vi "Teleop.vi"(10 "Match Info":T2={"Autonomous Elapsed Seconds"=0.0, "TeleOp Elapsed Seconds"=0.0, "Disabled Elapsed Seconds"=0.0, "Visited Autonomous"=FALSE, "Visited TeleOp"=FALSE, "Visited Disabled"=FALSE, "Autonomous Settings"={"Autonomous Style"=enum."Independent", "VI Refnum"=refnum}}, 11 "Call Context":T3) -> ()   [LabVIEW 2015]
doc: "This VI is called for each TeleOp packet received from the DS where the robot is not disabled. It is often used to read from the joysticks and update I/O or to update setpoints for timed control loops. It should complete and return within 20 milliseconds or it may miss DS packets."
uses:
  <vilib>/Rock Robotics/WPI/DriverStation/WPI_DriverStationDerivedRobotMode.ctl
  <vilib>/Rock Robotics/WPI/DriverStation/WPI_DriverStationMatch Info.ctl
  <vilib>/Rock Robotics/WPI/Utilities/WPI_GetSetVariantRefNum.vi
  <vilib>/Rock Robotics/Network Tables/NT Write Boolean Array.vi
  <vilib>/Rock Robotics/Network Tables/NT Write Numeric Array.vi
  <vilib>/Rock Robotics/Network Tables/NT Read Boolean.vi
  <vilib>/Rock Robotics/Network Tables/NT Read Number.vi
  Robot Global Data.vi
  <vilib>/Rock Robotics/Network Tables/NT Write Number.vi
  <vilib>/Rock Robotics/WPI/RobotDrive/WPI_RobotDriveArcadeDrive_Standard(NoSaturation).vi
panel:
  in  "Winch Lock":bool
  out "Ladder Up Start Time":u32
  in  "LadderStateMachine":i32
  out "Accelerations":T1
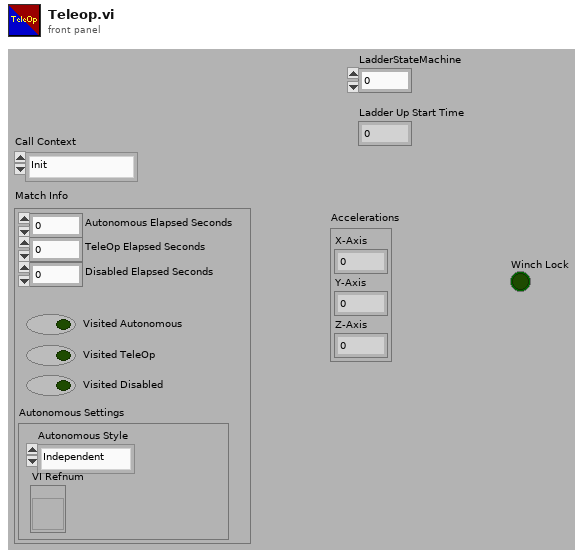
[diagram p1: front panel]
types:
  T1 = cluster{"X-Axis":dbl, "Y-Axis":dbl, "Z-Axis":dbl}
  T2 = typedef "WPI_DriverStationMatch Info.ctl" = cluster{"Autonomous Elapsed Seconds":dbl, "TeleOp Elapsed Seconds":dbl, "Disabled Elapsed Seconds":dbl, "Visited Autonomous":bool, "Visited TeleOp":bool, "Visited Disabled":bool, "Autonomous Settings":cluster{"Autonomous Style":enum16{"Iterative", "Independent"}, "VI Refnum":refnum<vi>}}
  T3 = typedef "WPI_DriverStationDerivedRobotMode.ctl" = enum16{"Init", "Execute", "Stop"}
  T4 = typedef "WPI_RobotDriveDevRef.ctl" = cluster{"DevStatus":errorcluster, "Motors[]":T5[], "Square Inputs":bool, "Max Output":dbl}
  T5 = typedef "WPI_MotorControlDeviceRef.ctl" = cluster{"DeviceStatus":errorcluster, "Type":T6, "PWM":cluster{"PWM Channel":T7, "DeadBand":T8}, "CAN":cluster{"Device Number":u8, "Control Mode":T9, "Semaphore":T10, "Max Vout":dbl, "TalonSRX Control Mode":T11}, "Invert":bool}
  T6 = typedef "WPI_MotorControlType.ctl" = enum16{"PWM", "CAN", "CANTalonSRX"}
  T7 = typedef "FPGA_DIOPWMChannel.ctl" = enum8{"PWM 0", "PWM 1", "PWM 2", "PWM 3", "PWM 4", "PWM 5", "PWM 6", "PWM 7", "PWM 8", "PWM 9", "PWM MXP 0", "PWM MXP 1", "PWM MXP 2", "PWM MXP 3", "PWM MXP 4", "PWM MXP 5", "PWM MXP 6", "PWM MXP 7", "PWM MXP 8", "PWM MXP 9", "Invalid"}
  T8 = typedef "WPI_PWMDeadband.ctl" = cluster{"Name":string, "maxPositivePwm":i32, "minPositivePwm":i32, "centerPwm":i32, "maxNegativePwm":i32, "minNegativePwm":i32, "angularRange":u16}
  T9 = typedef "WPI_CANJaguar_ControlMode.ctl" = enum8{"Percent VBus", "Current", "Speed", "Position", "Voltage"}
  T10 = typedef "Semaphore RefNum" = refnum<k1>
  T11 = typedef "WPI_CANTalonSRX_APIControlMode.ctl" = enum8{"Percent VBus", "Speed", "Position", "Slave", "Unchanged / Invalid", "Voltage Compensation", "Current", "Motion Profile"}
  T12 = typedef "WPI_JoystickDevRef.ctl" = cluster{"Device":T13}
  T13 = typedef "WPI_JoystickDeviceEnum.ctl" = enum16{"USB 0", "USB 1", "USB 2", "USB 3", "USB 4", "USB 5"}
  T14 = typedef "WPI_DigitalInputDevRef.ctl" = cluster{"DevStatus":errorcluster, "DIO Channel":T15}
  T15 = typedef "FPGA_DIOChannel.ctl" = enum8{"DIO 0", "DIO 1", "DIO 2", "DIO 3", "DIO 4", "DIO 5", "DIO 6", "DIO 7", "DIO 8", "DIO 9", "DIO MXP 0", "DIO MXP 1", "DIO MXP 2", "DIO MXP 3", "DIO MXP 4", "DIO MXP 5", "DIO MXP 6", "DIO MXP 7", "DIO MXP 8", "DIO MXP 9", "DIO MXP 10", "DIO MXP 11", "DIO MXP 12", "DIO MXP 13", "DIO MXP 14", "DIO MXP 15", "Invalid"}
  T16 = typedef "WPI_AccelerometerDevRef.ctl" = cluster{"DevStatus":errorcluster, "Scaling":T17, "Analog Channels":T18, "I2C Bus":T20, "SPI Bus":T21, "Accel Range":T22, "ADXL Axes":T23, "Handle":i32, "Device Address":u8, "Accel Type":enum16{"Analog", "ADXL345 I2C", "ADXL345 SPI", "Internal", "ADXL362 SPI"}}
  T17 = typedef "WPI_AccelerometerScaling.ctl" = cluster{"Gain (VoltsPerG)":dbl, "Center Voltage":dbl}
  T18 = typedef "WPI_AccelerometerAnalogChannels.ctl" = cluster{"X-Axis":T19, "Y-Axis":T19, "Z-Axis":T19}
  T19 = typedef "FPGA_AIChannel.ctl" = enum8{"AI 0", "AI 1", "AI 2", "AI 3", "AI MXP 0", "AI MXP 1", "AI MXP 2", "AI MXP 3", "Invalid"}
  T20 = typedef "i2c_bus.ctl" = enum16{"I2C On-Board", "I2C MXP", "Invalid"}
  T21 = typedef "spi_bus.ctl" = enum16{"SPI On-Board, CS0", "SPI On-Board, CS1", "SPI On-Board, CS2", "SPI On-Board, CS3", "SPI MXP", "Invalid"}
  T22 = typedef "ADXL345 Range.ctl" = u8
  T23 = typedef "WPI_AccelerometerADXL345 Axes.ctl" = cluster{"X-Axis":bool, "Y-Axis":bool, "Z-Axis":bool}
  T24 = typedef "WPI_EncoderDevRef.ctl" = cluster{"DevStatus":errorcluster, "EncoderIndex":T25, "CounterIndex":T26, "DistancePerCount":dbl, "Decoding Type":T27}
  T25 = typedef "FPGA_EncoderIdx.ctl" = enum8{"Enc 0", "Enc 1", "Enc 2", "Enc 3", "Enc 4", "Enc 5", "Enc 6", "Enc 7", "Invalid"}
  T26 = typedef "FPGA_CounterCtrSystemIndex.ctl" = enum8{"Ctr 0", "Ctr 1", "Ctr 2", "Ctr 3", "Ctr 4", "Ctr 5", "Ctr 6", "Ctr 7", "Invalid"}
  T27 = typedef "WPI_EncoderType.ctl" = enum16{"1x", "2x", "4x"}
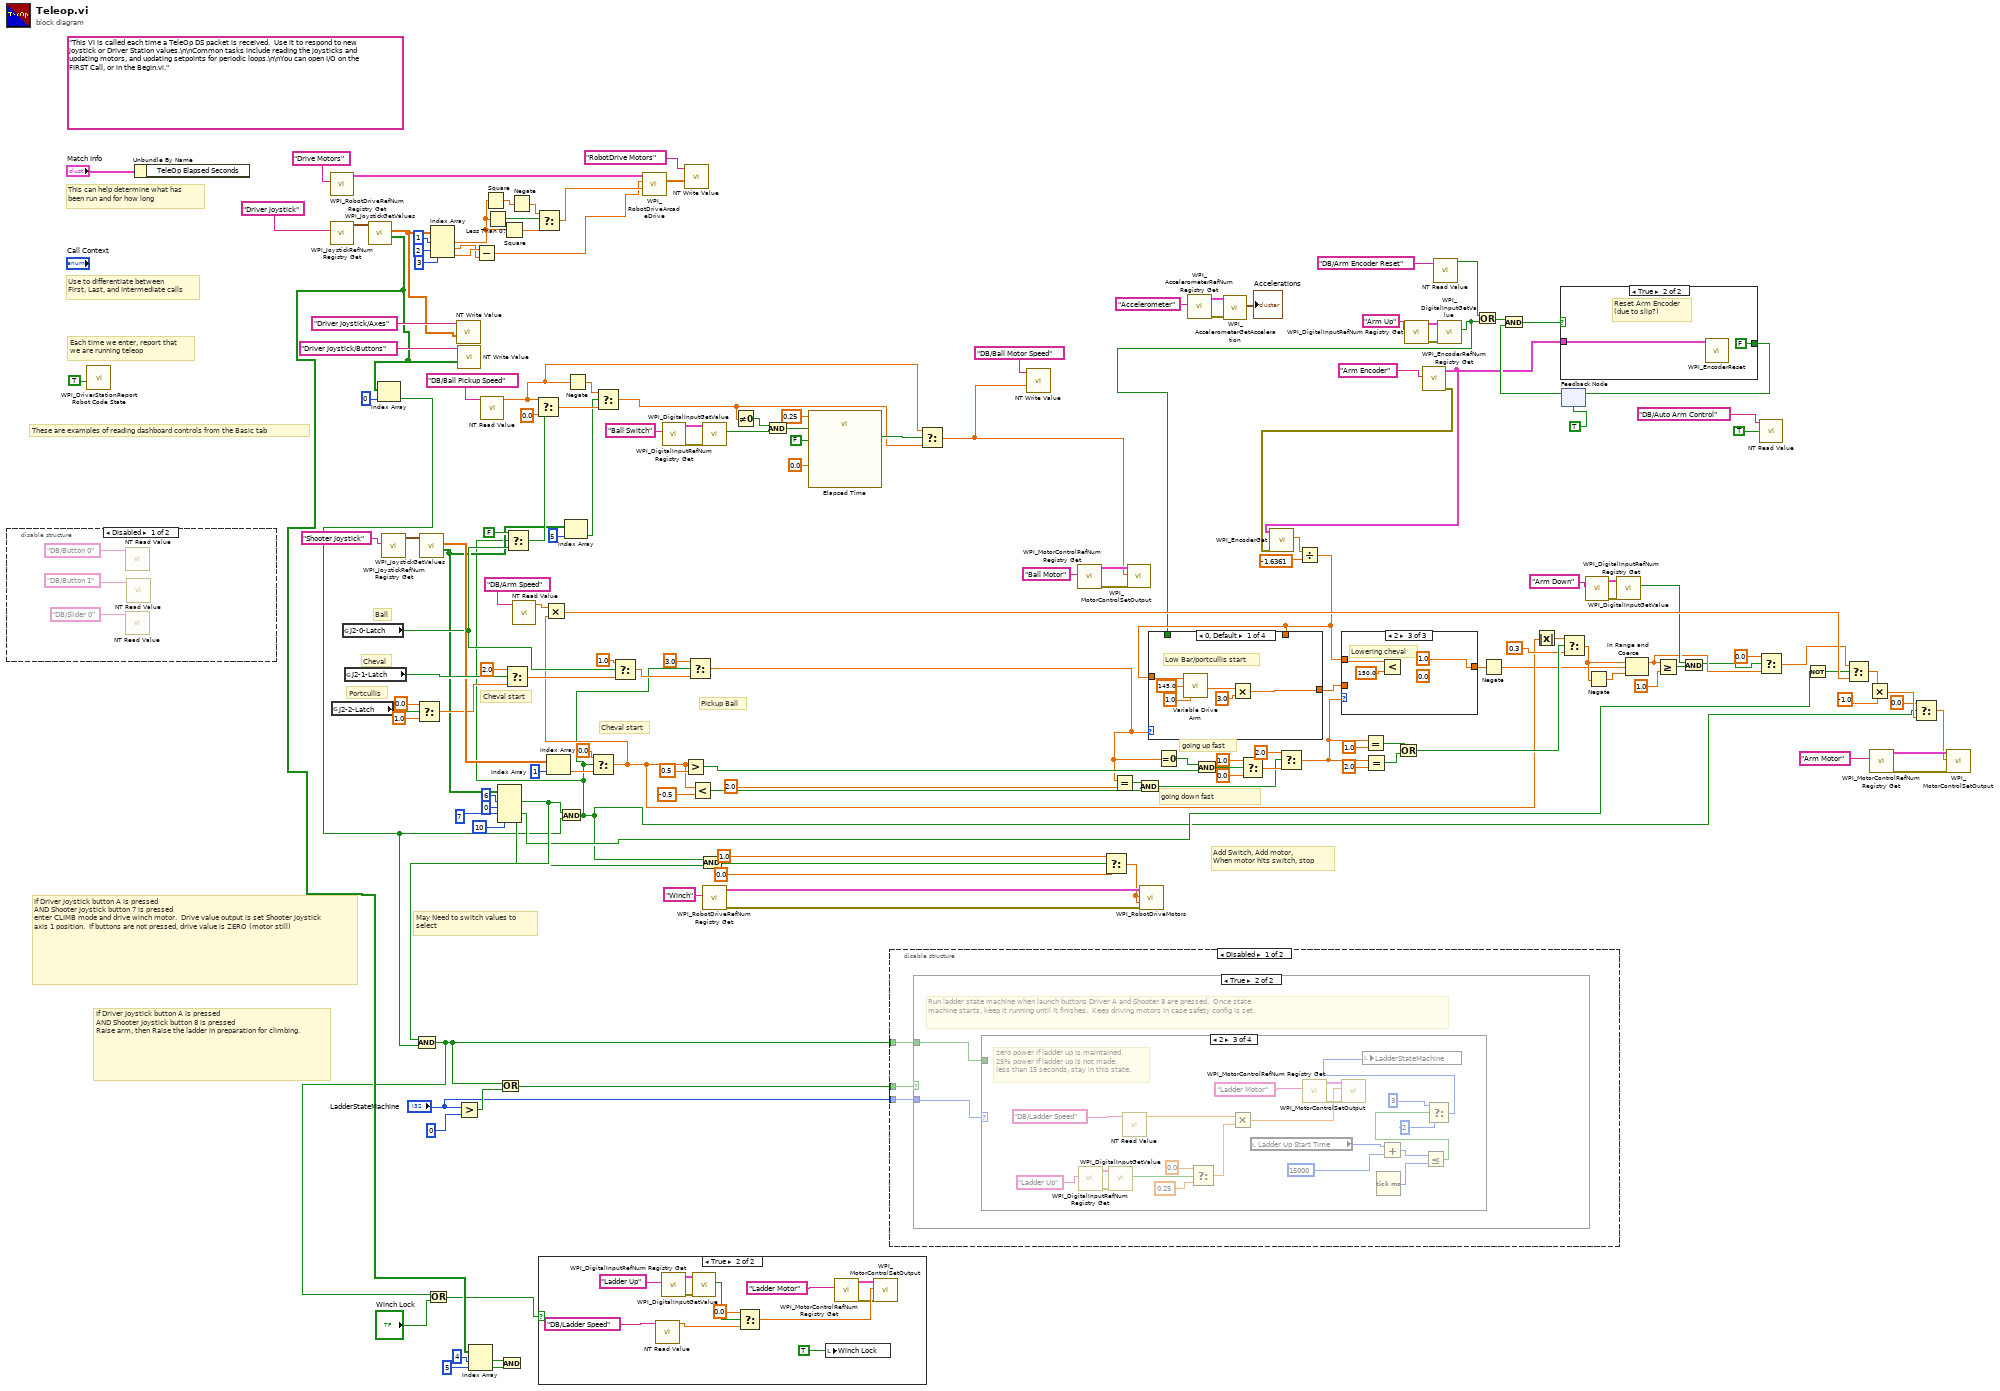
[diagram p0: block diagram]
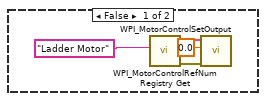
[diagram p2: hidden frame]
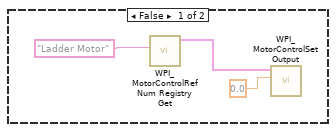
[diagram p3: hidden frame]
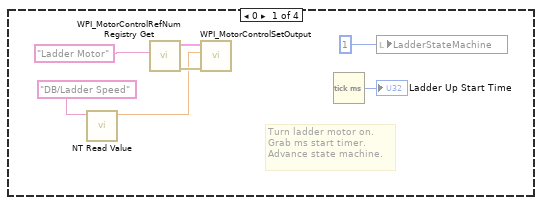
[diagram p4: hidden frame]
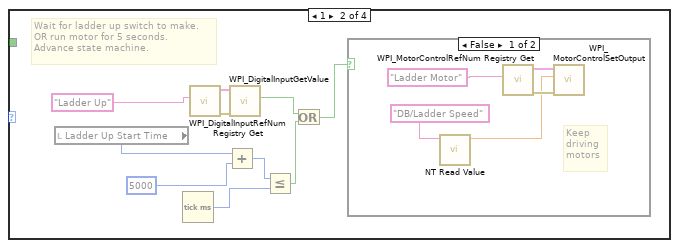
[diagram p5: hidden frame]
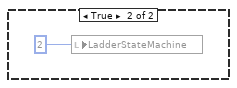
[diagram p6: hidden frame]
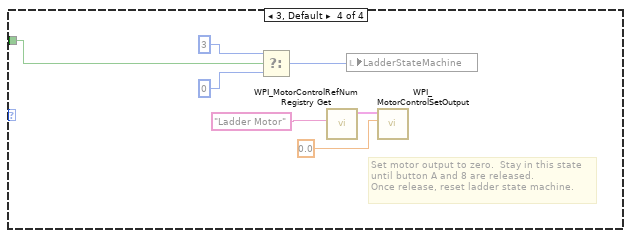
[diagram p7: hidden frame]
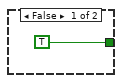
[diagram p9: hidden frame]
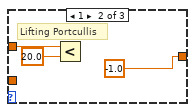
[diagram p12: hidden frame]
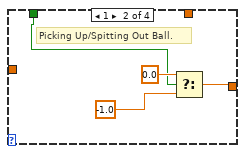
[diagram p13: hidden frame]
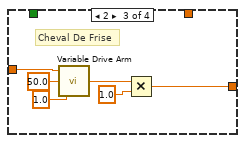
[diagram p14: hidden frame]
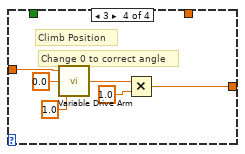
[diagram p15: hidden frame]
diagram:
  (unwired) "This VI is called each time a TeleOp DS packet is received.  Use it to respond to new joystick or Driver Station values.\n\nCommon tasks include reading the joysticks and updating motors, and updating setpoints for periodic loops.\n\nYou can open I/O on the FIRST Call, or in the Begin.vi."
  # "going up fast"
  # "going down fast"
  # "If Driver Joystick button A is pressed\nAND Shooter Joystick button 8 is pressed\nRaise arm, then Raise the ladder in preparation for climbing."
  # "If Driver Joystick button A is pressed\nAND Shooter Joystick button 7 is pressed\nenter CLIMB mode and drive winch motor.  Drive value output is set Shooter Joystick axis 1 position.  If buttons are not pressed, drive value is ZERO (motor still)"
  # "Add Switch, Add motor, \nWhen motor hits switch, stop"
  # "Portcullis"
  # "Ball"
  # "Cheval"
  # "May Need to switch values to \nselect"
  # "Cheval start"
  # "Pickup Ball"
  # "Cheval start"
  # "These are examples of reading dashboard controls from the Basic tab"
  # "Each time we enter, report that\nwe are running teleop"
  # "Use to differentiate between\nFirst, Last, and Intermediate calls"
  # "This can help determine what has\nbeen run and for how long"
  n1 = disable-structure shown="Disabled" {
    frame Disabled {
      n2 = call-poly <vilib>:"NT Read Value.vi"("Name"="DB/Button 0" ("refnum name")) -> ("Boolean"=w169:bool)  [unwired: 9 in, 1 out]
      n3 = call-poly <vilib>:"NT Read Value.vi"("Name"="DB/Slider 0" ("refnum name")) -> ("Numeric"=w171:dbl)  [unwired: 9 in, 1 out]
      n4 = call-poly <vilib>:"NT Read Value.vi"("Name"="DB/Button 1" ("refnum name")) -> ("Boolean"=w170:bool)  [unwired: 9 in, 1 out]
    }
    frame Enabled {
    }
  }
  n5 = call <vilib>:"WPI_DriverStationReport Robot Code State.vi"("TeleOp"=TRUE ("Autonomous")) -> ()  [unwired: 10 in, 1 out]
  n6 = Unbundle By Name("Match Info") -> ()  [unwired: 1 out]
  n7 = call <vilib>:"WPI_RobotDriveRefNum Registry Get.vi"("refnum name"="Drive Motors") -> ("RobotDriveDevRef"=w165:T4)  [unwired: 1 in, 9 out]
  n8 = call <vilib>:"WPI_JoystickRefNum Registry Get.vi"("refnum name"="Driver Joystick") -> ("JoystickDevRef"=w163:T12)  [unwired: 1 in, 9 out]
  n9 = global read "Robot Global Data.vi" "J2-2-Latch"() -> (w88:bool)
  n10 = global read "Robot Global Data.vi" "J2-0-Latch"() -> (w84:bool)
  n11 = global read "Robot Global Data.vi" "J2-1-Latch"() -> (w141:bool)
  n12 = call <vilib>:"WPI_JoystickGetValues.vi"("JoystickDevRef"=w163) -> ("Buttons"=w32:bool[], "Axes"=w153:dbl[])  [unwired: 6 in, 3 out]
  n13 = Index Array(array=w32, index=0) -> (element=w31:bool)
  n14 = call <vilib>:"WPI_JoystickRefNum Registry Get.vi"("refnum name"="Shooter Joystick") -> ("JoystickDevRef"=w152:T12)  [unwired: 1 in, 9 out]
  n15 = Select(t=0.0, s=w88, f=1.0) -> (s? t:f=w89:dbl)
  n16 = call <vilib>:"WPI_JoystickGetValues.vi"("JoystickDevRef"=w152) -> ("Buttons"=w56:bool[], "Axes"=w117:dbl[])  [unwired: 6 in, 3 out]
  n17 = Index Array(array=w153, index #1=1 ("index"), index #2=2 ("index"), index #3=3 ("index")) -> (element #1=w113:dbl, element #2=w110:dbl, element #3=w111:dbl)
  n18 = call-poly <vilib>:"NT Write Value.vi"("Numeric Array"=w153, "Name"="Driver Joystick/Axes") -> ()  [unwired: 9 in, 1 out]
  n19 = call-poly <vilib>:"NT Write Value.vi"("Boolean Array"=w32, "Name"="Driver Joystick/Buttons") -> ()  [unwired: 9 in, 1 out]
  n20 = Greater?(x="LadderStateMachine", y=0) -> (0:w69:bool)
  n21 = Index Array(array=w32, index #1=4 ("index"), index #2=5 ("index")) -> (element #1=w27:bool, element #2=w28:bool)
  n22 = Subtract(x=w111, y=w110) -> (x-y=w109:dbl)
  n23 = call-poly <vilib>:"NT Read Value.vi"("Name"="DB/Ball Pickup Speed") -> ("Numeric"=w7:dbl)  [unwired: 9 in, 1 out]
  n24 = Square(x=w113) -> (x^2=w157:dbl)
  n25 = Less Than 0?(x=w113) -> (x < 0?=w159:bool)
  n26 = Index Array(array=w56, index #1=6 ("index"), index #2=0 ("index"), index #3=7 ("index"), index #4=10 ("index")) -> (element #1=w66:bool, element #3=w48:bool, element #4=w36:bool)  [unwired: 1 out]
  n27 = And(x=w66, y=w31) -> (x .and. y?=w25:bool)
  n28 = Or(x=w25, y="Winch Lock") -> (x .or. y?=w14:bool)
  n29 = Or(x=w25, y=w69) -> (x .or. y?=w68:bool)
  n30 = And(x=w27, y=w28) -> ()  [unwired: 1 out]
  n31 = Square(x=w113) -> (x^2=w156:dbl)
  n32 = Select(t=2.0, s=w141, f=w89) -> (s? t:f=w142:dbl)
  n33 = Negate(x=w157) -> (-x=w158:dbl)
  n34 = call-poly <vilib>:"NT Read Value.vi"("Name"="DB/Arm Speed") -> ("Numeric"=w78:dbl)  [unwired: 9 in, 1 out]
  n35 = Select(t=w158, s=w159, f=w156) -> (s? t:f=w116:dbl)
  n36 = case shown="True" w14 {
    frame False {
      n37 = call <vilib>:"WPI_MotorControlRefNum Registry Get.vi"("refnum name"="Ladder Motor") -> ("error out"=w176:errorcluster, "MotorControlDevRef"=w178:T5)  [unwired: 9 in]
      n38 = call <vilib>:"WPI_MotorControlSetOutput.vi"("error in (no error)"=w176, "Output"=0.0, "MotorControlDevRef"=w178) -> ()  [unwired: 6 in, 3 out]
    }
    frame True {
      n39 = call-poly <vilib>:"NT Read Value.vi"("Name"="DB/Ladder Speed") -> ("Numeric"=w184:dbl)  [unwired: 9 in, 1 out]
      n40 = call <vilib>:"WPI_DigitalInputRefNum Registry Get.vi"("refnum name"="Ladder Up") -> ("error out"=w190:errorcluster, "DigitalInputDevRef"=w188:T14)  [unwired: 9 in]
      n41 = call <vilib>:"WPI_DigitalInputGetValue.vi"("error in (no error)"=w190, "DigitalInputDevRef"=w188) -> ("Value"=w187:bool)  [unwired: 7 in, 2 out]
      n42 = Select(t=0.0, s=w187, f=w184) -> (s? t:f=w181:dbl)
      n43 = local write "Winch Lock"(TRUE) -> ()
      n44 = call <vilib>:"WPI_MotorControlRefNum Registry Get.vi"("refnum name"="Ladder Motor") -> ("error out"=w180:errorcluster, "MotorControlDevRef"=w183:T5)  [unwired: 9 in]
      n45 = call <vilib>:"WPI_MotorControlSetOutput.vi"("error in (no error)"=w180, "Output"=w181, "MotorControlDevRef"=w183) -> ()  [unwired: 6 in, 3 out]
    }
  }
  n46 = Index Array(array=w117, index=1) -> (element=w108:dbl)
  n47 = And(x=w66, y=w31) -> (x .and. y?=w38:bool)
  n48 = Select(t=FALSE, s=w38, f=w84) -> (s? t:f=w85:bool)
  n49 = Select(t=w7, s=w85, f=0.0) -> (s? t:f=w58:dbl)
  n50 = Index Array(array=w56, index=5) -> (element=w54:bool)
  n51 = Negate(x=w7) -> (-x=w57:dbl)
  n52 = Select(t=0.0, s=w38, f=w108) -> (s? t:f=w79:dbl)
  n53 = Multiply(x=w78, y=w79) -> (x*y=w74:dbl)
  n54 = Select(t=w57, s=w54, f=w58) -> (s? t:f=w6:dbl)
  n55 = Select(t=1.0, s=w84, f=w142) -> (s? t:f=w93:dbl)
  n56 = call-poly <vilib>:"WPI_RobotDriveArcadeDrive.vi"("Y axis value"=w116, "X axis value"=w109, "RobotDriveDevRef"=w165) -> ("Motor Values"=w162:dbl[])  [unwired: 6 in, 2 out]
  n57 = call <vilib>:"WPI_DigitalInputRefNum Registry Get.vi"("refnum name"="Ball Switch") -> ("error out"=w9:errorcluster, "DigitalInputDevRef"=w10:T14)  [unwired: 9 in]
  n58 = Greater?(x=w79, y=0.5) -> (0:w137:bool)
  n59 = call-poly <vilib>:"NT Write Value.vi"("Numeric Array"=w162, "Name"="RobotDrive Motors") -> ()  [unwired: 9 in, 1 out]
  n60 = Select(t=3.0, s=w38, f=w93) -> (s? t:f=w94:dbl)
  n61 = Less?(x=w79, y=-0.5) -> (x < y?=w131:bool)
  n62 = And(x=w38, y=w36) -> (x .and. y?=w39:bool)
  n63 = call <vilib>:"WPI_DigitalInputGetValue.vi"("error in (no error)"=w9, "DigitalInputDevRef"=w10) -> ("Value"=w3:bool)  [unwired: 7 in, 2 out]
  n64 = call <vilib>:"WPI_RobotDriveRefNum Registry Get.vi"("refnum name"="Winch") -> ("error out"=w123:errorcluster, "RobotDriveDevRef"=w122:T4)  [unwired: 9 in]
  n65 = Not Equal To 0?(x=w6) -> (x != 0?=w5:bool)
  n66 = And(x=w5, y=w3) -> (x .and. y?=w4:bool)
  n67 = call "Elapsed Time"("Time Target (s)"=0.25, "Reset"=w4, "Auto Reset"=FALSE, "Set Start Time (s)"=0.0) -> ("Time has Elapsed"=w11:bool)  [unwired: 8 in, 7 out]
  n68 = disable-structure shown="Disabled" {
    disable-tunnel: w68 -> [w193 _]
    disable-tunnel: "LadderStateMachine" -> [w192 _]
    disable-tunnel: w25 -> [w191 _]
    frame Disabled {
      n69 = case shown="True" w193 {
        tunnel: w192 -> [_ w198]
        tunnel: w191 -> [_ w197]
        frame False {
          n70 = call <vilib>:"WPI_MotorControlRefNum Registry Get.vi"("refnum name"="Ladder Motor") -> ("MotorControlDevRef"=w194:T5)  [unwired: 9 in, 1 out]
          n71 = call <vilib>:"WPI_MotorControlSetOutput.vi"("Output"=0.0, "MotorControlDevRef"=w194) -> ()  [unwired: 7 in, 3 out]
        }
        frame True {
          # "Run ladder state machine when launch buttons Driver A and Shooter 8 are pressed.  Once state\nmachine starts, keep it running until it finishes.  Keep driving motors in case safety config is set."
          n72 = case shown="2" w198 {
            tunnel: w197 -> [_ _ _ w247]
            frame 0 {
              # "Turn ladder motor on.\nGrab ms start timer.\nAdvance state machine."
              n73 = call-poly <vilib>:"NT Read Value.vi"("Name"="DB/Ladder Speed") -> ("Numeric"=w201:dbl)  [unwired: 9 in, 1 out]
              n74 = call <vilib>:"WPI_MotorControlRefNum Registry Get.vi"("refnum name"="Ladder Motor") -> ("error out"=w205:errorcluster, "MotorControlDevRef"=w204:T5)  [unwired: 9 in]
              n75 = call <vilib>:"WPI_MotorControlSetOutput.vi"("error in (no error)"=w205, "Output"=w201, "MotorControlDevRef"=w204) -> ()  [unwired: 6 in, 3 out]
              n76 = Tick Count (ms)() -> (millisecond timer value=→"Ladder Up Start Time":u32)
              n77 = local write "LadderStateMachine"(1 ("LadderStateMachine")) -> ()
            }
            frame 1 {
              # "Wait for ladder up switch to make.\nOR run motor for 5 seconds.\nAdvance state machine."
              n78 = local read "Ladder Up Start Time"() -> (w211:u32)
              n79 = Tick Count (ms)() -> (millisecond timer value=w209:u32)
              n80 = call <vilib>:"WPI_DigitalInputRefNum Registry Get.vi"("refnum name"="Ladder Up") -> ("error out"=w215:errorcluster, "DigitalInputDevRef"=w213:T14)  [unwired: 9 in]
              n81 = Add(x=w211, y=u32 5000) -> (x+y=w210:u32)
              n82 = call <vilib>:"WPI_DigitalInputGetValue.vi"("error in (no error)"=w215, "DigitalInputDevRef"=w213) -> ("Value"=w206:bool)  [unwired: 7 in, 2 out]
              n83 = Less Or Equal?(x=w210, y=w209) -> (x <= y?=w207:bool)
              n84 = Or(x=w206, y=w207) -> (x .or. y?=w208:bool)
              n85 = case shown="False" w208 {
                frame False {
                  # "Keep\ndriving \nmotors"
                  n86 = call-poly <vilib>:"NT Read Value.vi"("Name"="DB/Ladder Speed") -> ("Numeric"=w216:dbl)  [unwired: 9 in, 1 out]
                  n87 = call <vilib>:"WPI_MotorControlRefNum Registry Get.vi"("refnum name"="Ladder Motor") -> ("error out"=w220:errorcluster, "MotorControlDevRef"=w219:T5)  [unwired: 9 in]
                  n88 = call <vilib>:"WPI_MotorControlSetOutput.vi"("error in (no error)"=w220, "Output"=w216, "MotorControlDevRef"=w219) -> ()  [unwired: 6 in, 3 out]
                }
                frame True {
                  n89 = local write "LadderStateMachine"(2 ("LadderStateMachine")) -> ()
                }
              }
            }
            frame 2 {
              # "zero power if ladder up is maintained.\n25% power if ladder up is not made.\nless than 15 seconds, stay in this state."
              n90 = call <vilib>:"WPI_DigitalInputRefNum Registry Get.vi"("refnum name"="Ladder Up") -> ("error out"=w236:errorcluster, "DigitalInputDevRef"=w234:T14)  [unwired: 9 in]
              n91 = call <vilib>:"WPI_DigitalInputGetValue.vi"("error in (no error)"=w236, "DigitalInputDevRef"=w234) -> ("Value"=w233:bool)  [unwired: 7 in, 2 out]
              n92 = call-poly <vilib>:"NT Read Value.vi"("Name"="DB/Ladder Speed") -> ("Numeric"=w238:dbl)  [unwired: 9 in, 1 out]
              n93 = Select(t=0.0, s=w233, f=0.25 ("y")) -> (s? t:f=w230:dbl)
              n94 = Multiply(x=w238, y=w230) -> (x*y=w237:dbl)
              n95 = local read "Ladder Up Start Time"() -> (w228:u32)
              n96 = call <vilib>:"WPI_MotorControlRefNum Registry Get.vi"("refnum name"="Ladder Motor") -> ("error out"=w242:errorcluster, "MotorControlDevRef"=w241:T5)  [unwired: 9 in]
              n97 = call <vilib>:"WPI_MotorControlSetOutput.vi"("error in (no error)"=w242, "Output"=w237, "MotorControlDevRef"=w241) -> ()  [unwired: 6 in, 3 out]
              n98 = Tick Count (ms)() -> (millisecond timer value=w226:u32)
              n99 = Add(x=w228, y=u32 15000) -> (x+y=w227:u32)
              n100 = Less Or Equal?(x=w227, y=w226) -> (x <= y?=w225:bool)
              n101 = Select(t=3 ("LadderStateMachine"), s=w225, f=2) -> (s? t:f=w222:i32)
              n102 = local write "LadderStateMachine"(w222) -> ()
            }
            frame 3, Default {
              # "Set motor output to zero.  Stay in this state\nuntil button A and 8 are released.\nOnce release, reset ladder state machine."
              n103 = Select(t=3 ("y"), s=w247, f=0 ("y")) -> (s? t:f=w246:i32)
              n104 = call <vilib>:"WPI_MotorControlRefNum Registry Get.vi"("refnum name"="Ladder Motor") -> ("MotorControlDevRef"=w245:T5)  [unwired: 9 in, 1 out]
              n105 = local write "LadderStateMachine"(w246) -> ()
              n106 = call <vilib>:"WPI_MotorControlSetOutput.vi"("Output"=0.0, "MotorControlDevRef"=w245) -> ()  [unwired: 7 in, 3 out]
            }
          }
        }
      }
    }
    frame Enabled {
    }
  }
  n107 = Select(t=w7, s=w11, f=w6) -> (s? t:f=w1:dbl)
  n108 = call-poly <vilib>:"NT Write Value.vi"("Numeric"=w1, "Name"="DB/Ball Motor Speed") -> ()  [unwired: 9 in, 1 out]
  n109 = call <vilib>:"WPI_MotorControlRefNum Registry Get.vi"("refnum name"="Ball Motor") -> ("error out"=w145:errorcluster, "MotorControlDevRef"=w146:T5)  [unwired: 9 in]
  n110 = Select(t=1.0, s=w39, f=0.0) -> (s? t:f=w40:dbl)
  n111 = Equal?(x=w94, y=2.0) -> (x = y?=w130:bool)
  n112 = call <vilib>:"WPI_MotorControlSetOutput.vi"("error in (no error)"=w145, "Output"=w1, "MotorControlDevRef"=w146) -> ()  [unwired: 6 in, 3 out]
  n113 = And(x=w130, y=w131) -> (x .and. y?=w127:bool)
  n114 = call <vilib>:"WPI_RobotDriveMotors.vi"("error in (no error)"=w123, "RightSpeed"=w40, "LeftSpeed"=w40, "RobotDriveDevRef"=w122) -> ()  [unwired: 5 in, 3 out]
  n115 = Equal To 0?(x=w94) -> (x = 0?=w140:bool)
  n116 = call <vilib>:"WPI_AccelerometerRefNum Registry Get.vi"("refnum name"="Accelerometer") -> ("error out"=w120:errorcluster, "AccelerometerDevRef"=w119:T16)  [unwired: 9 in]
  n117 = And(x=w140, y=w137) -> (x .and. y?=w136:bool)
  n118 = call <vilib>:"WPI_AccelerometerGetAcceleration.vi"("error in"=w120, "AccelerometerDevRef"=w119) -> ("Accelerations"=→"Accelerations":T1)  [unwired: 7 in, 2 out]
  n119 = Select(t=1.0, s=w136, f=0.0) -> (s? t:f=w128:dbl)
  n120 = Select(t=2.0, s=w127, f=w128) -> (s? t:f=w105:dbl)
  n121 = Equal?(x=w105, y=1.0) -> (x = y?=w103:bool)
  n122 = Equal?(x=w105, y=2.0) -> (x = y?=w102:bool)
  n123 = Or(x=w103, y=w102) -> (x .or. y?=w101:bool)
  n124 = call <vilib>:"WPI_DigitalInputRefNum Registry Get.vi"("refnum name"="Arm Up") -> ("error out"=w43:errorcluster, "DigitalInputDevRef"=w42:T14)  [unwired: 9 in]
  n125 = call <vilib>:"WPI_EncoderRefNum Registry Get.vi"("refnum name"="Arm Encoder") -> ("error out"=w63:errorcluster, "EncoderDevRef"=w64:T24)  [unwired: 9 in]
  n126 = call <vilib>:"WPI_EncoderGet.vi"("error in (no error)"=w63, "EncoderDevRef"=w64) -> ("Distance"=w61:dbl)  [unwired: 4 in, 5 out]
  n127 = Divide(x=w61, y=-1.6361 ("Arm Calibration")) -> (x/y=w60:dbl)
  n128 = call-poly <vilib>:"NT Read Value.vi"("Name"="DB/Arm Encoder Reset") -> ("Boolean"=w45:bool)  [unwired: 9 in, 1 out]
  n129 = call <vilib>:"WPI_DigitalInputGetValue.vi"("error in (no error)"=w43, "DigitalInputDevRef"=w42) -> ("Value"=w41:bool)  [unwired: 7 in, 2 out]
  n130 = case shown="0, Default" w94 {
    tunnel: w60 -> [w255 _ w260 w266]
    tunnel: [w252 w259 w261 w267] -> w133
    tunnel: w60 -> [_ _ _ _]
    tunnel: w41 -> [_ w256 _ _]
    frame 0, Default {
      # "Low Bar/portcullis start"
      n131 = call "Variable Drive Arm.vi"("Max Speed"=1.0, "Wanted Angle"=145.0, "Encoder"=w255) -> ("Motor Controller"=w251:dbl)
      n132 = Multiply(x=w251, y=3.0) -> (x*y=w252:dbl)
    }
    frame 1 {
      # "Picking Up/Spitting Out Ball."
      n133 = Select(t=0.0, s=w256, f=-1.0) -> (s? t:f=w259:dbl)
    }
    frame 2 {
      # "Cheval De Frise"
      n134 = call "Variable Drive Arm.vi"("Max Speed"=1.0, "Wanted Angle"=50.0, "Encoder"=w260) -> ("Motor Controller"=w263:dbl)
      n135 = Multiply(x=w263, y=1.0) -> (x*y=w261:dbl)
    }
    frame 3 {
      # "Change 0 to correct angle"
      # "Climb Position"
      n136 = call "Variable Drive Arm.vi"("Max Speed"=1.0, "Wanted Angle"=0.0, "Encoder"=w266) -> ("Motor Controller"=w269:dbl)
      n137 = Multiply(x=w269, y=1.0) -> (x*y=w267:dbl)
    }
  }
  n138 = case shown="2" w105 {
    tunnel: w60 -> [_ w275 w278]
    tunnel: [w272 -1.0 ("f") 1.0 ("t")] -> w97
    tunnel: w133 -> [w272 _ _]
    frame 0, Default {
    }
    frame 1 {
      # "Lifting Portcullis"
      n139 = Less?(x=w275, y=20.0) -> ()  [unwired: 1 out]
    }
    frame 2 {
      (unwired) 0.0 ("f")
      # "Lowering cheval"
      n140 = Less?(x=w278, y=150.0) -> ()  [unwired: 1 out]
    }
  }
  n141 = Or(x=w45, y=w41) -> (x .or. y?=w46:bool)
  n142 = Negate(x=w97) -> (-x=w53:dbl)
  n143 = Absolute Value(x=w79) -> (abs(x)=w100:dbl)
  n144 = feedback #1(TRUE) -> (w72:bool)
  n145 = And(x=w46, y=w72) -> (x .and. y?=w59:bool)
  n146 = case shown="True" w59 {
    tunnel: [TRUE FALSE] -> w71
    tunnel: w64 -> [_ w280]
    frame False {
    }
    frame True {
      # "Reset Arm Encoder\n(due to slip?)"
      n147 = call <vilib>:"WPI_EncoderReset.vi"("EncoderDevRef"=w280) -> ()  [unwired: 9 in, 2 out]
    }
  }
  n148 = feedback-in #1(w71) -> ()
  n149 = Select(t=w100, s=w101, f=0.3) -> (s? t:f=w98:dbl)
  n150 = call <vilib>:"WPI_DigitalInputRefNum Registry Get.vi"("refnum name"="Arm Down") -> ("error out"=w22:errorcluster, "DigitalInputDevRef"=w21:T14)  [unwired: 9 in]
  n151 = Negate(x=w98) -> (-x=w99:dbl)
  n152 = call <vilib>:"WPI_DigitalInputGetValue.vi"("error in (no error)"=w22, "DigitalInputDevRef"=w21) -> ("Value"=w19:bool)  [unwired: 7 in, 2 out]
  n153 = In Range and Coerce(upper limit=w98, x=w53, lower limit=w99) -> (coerced(x)=w17:dbl)  [unwired: 1 out]
  n154 = Greater Or Equal?(x=w17, y=1.0 ("x")) -> (x >= y?=w23:bool)
  n155 = And(x=w19, y=w23) -> (x .and. y?=w15:bool)
  n156 = call-poly <vilib>:"NT Read Value.vi"("Default Value"=TRUE, "Name"="DB/Auto Arm Control") -> ()  [unwired: 8 in, 2 out]
  n157 = Select(t=0.0, s=w15, f=w17) -> (s? t:f=w18:dbl)
  n158 = Not(x=w48) -> (.not. x?=w47:bool)
  n159 = Select(t=w18, s=w47, f=w74) -> (s? t:f=w107:dbl)
  n160 = Multiply(x=w107, y=-1.0) -> (x*y=w51:dbl)
  n161 = call <vilib>:"WPI_MotorControlRefNum Registry Get.vi"("refnum name"="Arm Motor") -> ("error out"=w148:errorcluster, "MotorControlDevRef"=w149:T5)  [unwired: 9 in]
  n162 = Select(t=0.0, s=w38, f=w51) -> (s? t:f=w52:dbl)
  n163 = call <vilib>:"WPI_MotorControlSetOutput.vi"("error in (no error)"=w148, "Output"=w52, "MotorControlDevRef"=w149) -> ()  [unwired: 6 in, 3 out]
